vi "FileIO-Get Format ID.vi"(0 "refnum":refnum<file>, 11 "error in (no error)":errorcluster) -> (4 "refnum out":refnum<file>, 8 "Format ID":i32, 15 "error out":errorcluster)   [LabVIEW 2015]
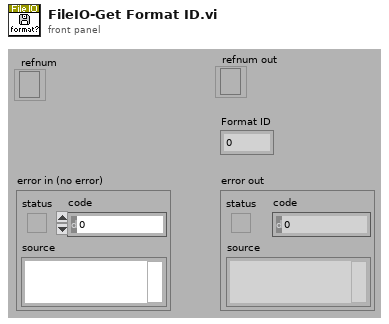
[diagram p1: front panel]
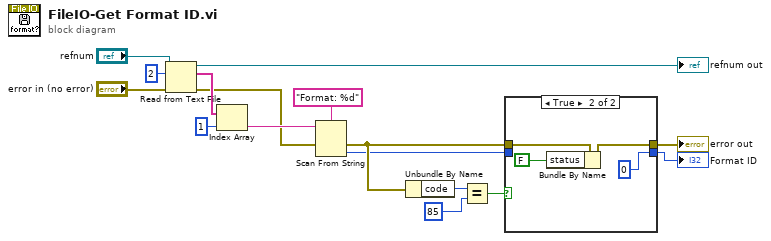
[diagram p0: block diagram]
diagram:
  n1 = Read from Text File(file (use dialog)="refnum", count=2, error in="error in (no error)") -> (refnum out=→"refnum out":refnum<file>, text=w15:string[], error out=w8:errorcluster)  [unwired: 1 in, 1 out]
  n2 = Index Array(array=w15, index=1) -> (element=w10:string)
  n3 = Scan From String(format string="Format: %d", input string=w10, error in=w8) -> (error out=w4:errorcluster, output 1=w3:i32)  [unwired: 2 in, 2 out]
  n4 = Unbundle By Name(w4) -> ("code"=w7:i32)
  n5 = Equal?(x=w7, y=85) -> (x = y?=w5:bool)
  n6 = case shown="True" w5 {
    tunnel: w4 -> [w18 w21]
    tunnel: w3 -> [w17 _]
    tunnel: [w18 w20] -> w2
    tunnel: [w17 0] -> w1
    frame False {
    }
    frame True {
      n7 = Bundle By Name(cluster=w21, "status"=FALSE) -> (w20:errorcluster)
    }
  }
  "error out" <- w2
  "Format ID" <- w1
